vi "nanocal -- nuclear schottky fit V4.vi"() -> ()   [LabVIEW 2020] (continued)
              n311 = Number To Fractional String(number=w690, precision (6)=i16 3) -> (F-format string=w691:string)  [unwired: 2 in]
              n312 = Insert Into Map(map in=w694, key=w692, value=w690) -> (map out=w693:map{i32, dbl})  [unwired: 2 out]
            }
            "T lookup" <- w654
            n313 = for {
              shift-right: [w687] -> w649
              shift-left: w650 -> [w688]
              tunnel: [w685] -> w647 mode=indexing
              tunnel: w648 -> [w684] mode=indexing
              i -> [w686]
              n314 = Number To Decimal String(number=w684) -> (decimal integer string=w685:string)  [unwired: 1 in]
              n315 = Insert Into Map(map in=w688, key=w686, value=w684) -> (map out=w687:map{i32, dbl})  [unwired: 2 out]
            }
            "Side lookup" <- w649
            n316 = local read "Set of Change"() -> (w644:set{dbl})
            n317 = property on="select side (8S|4R)" class="Ring (strict)"("Strings []"=w647) -> ()  [unwired: 2 in, 2 out]
            n318 = for {
              shift-right: [w682] -> w645
              shift-left: w646 -> [w683]
              tunnel: [w680] -> w643 mode=indexing
              tunnel: w644 -> [w679] mode=indexing
              i -> [w681]
              n319 = Number To Decimal String(number=w679) -> (decimal integer string=w680:string)  [unwired: 1 in]
              n320 = Insert Into Map(map in=w683, key=w681, value=w679) -> (map out=w682:map{i32, dbl})  [unwired: 2 out]
            }
            "change lookup" <- w645
            n321 = local read "temps&degs"() -> (w660:map{string, map{T5, dbl}})
            n322 = local read "X selector"() -> (w659:T5)
            n323 = property on="select T (K)" class="Ring (strict)"("Strings []"=w653) -> ()  [unwired: 2 in, 2 out]
            n324 = for {
              tunnel: [w715] -> w670 mode=indexing
              tunnel: [w719] -> w668 mode=indexing
              tunnel: [w716] -> w672 mode=indexing
              tunnel: w659 -> [w720]
              tunnel: w640 -> [w718] mode=indexing
              tunnel: w660 -> [w717]
              n325 = Unbundle(w718) -> (w715:string, w716:string)
              n326 = Look In Map(map=w717, key=w716) -> (value=w721:map{T5, dbl})  [unwired: 1 in, 1 out]
              n327 = Look In Map(map=w721, key=w720) -> (value=w719:dbl)  [unwired: 1 in, 1 out]
            }
            n328 = property on="select set (1T|2B)" class="Ring (strict)"("Strings []"=w643) -> ()  [unwired: 2 in, 2 out]
            n329 = local read "Set of θ's"() -> (w658:set{dbl})
            n330 = local read "Set of B's"() -> (w657:set{dbl})
            n331 = for {
              shift-right: [w707] -> w667
              shift-left: w662 -> [w708]
              tunnel: [w705] -> w666 mode=indexing
              tunnel: w657 -> [w704] mode=indexing
              i -> [w706]
              n332 = Number To Fractional String(number=w704, precision (6)=i16 3) -> (F-format string=w705:string)  [unwired: 2 in]
              n333 = Insert Into Map(map in=w708, key=w706, value=w704) -> (map out=w707:map{i32, dbl})  [unwired: 2 out]
            }
            "B lookup" <- w667
            n334 = for {
              shift-right: [w713] -> w665
              shift-left: w661 -> [w714]
              tunnel: [w711] -> w664 mode=indexing
              tunnel: w658 -> [w710] mode=indexing
              i -> [w712]
              n335 = Number To Fractional String(number=w710, precision (6)=i16 3) -> (F-format string=w711:string)  [unwired: 2 in]
              n336 = Insert Into Map(map in=w714, key=w712, value=w710) -> (map out=w713:map{i32, dbl})  [unwired: 2 out]
            }
            "θ lookup" <- w665
            n337 = call "array - sorted inexes.vi"("x"=w668) -> ("index array"=w669:i32[])  [unwired: 9 in, 1 out]
            n338 = property on="select B (T)" class="Ring (strict)"("Strings []"=w666) -> ()  [unwired: 2 in, 2 out]
            n339 = property on="select θ (deg)" class="Ring (strict)"("Strings []"=w664) -> ()  [unwired: 2 in, 2 out]
            n340 = for {
              tunnel: w669 -> [w699] mode=indexing
              tunnel: w670 -> [w702]
              tunnel: [w701] -> w671 mode=indexing
              tunnel: w672 -> [w700]
              shift-right: [w695] -> w673
              shift-left: w663 -> [w698]
              i -> [w697]
              n341 = Index Array(array=w702, index=w699) -> (element=w701:string)
              n342 = Index Array(array=w700, index=w699) -> (element=w696:string)
              n343 = Insert Into Map(map in=w698, key=w697, value=w696) -> (map out=w695:map{i32, string})  [unwired: 2 out]
            }
            "filesnames lookup" <- w673
            n344 = property on="filenames" class="Ring (strict)"("Strings []"=w671) -> ()  [unwired: 2 in, 2 out]
          }
          frame "action: update constrained file selector" {
            (unwired) ""
            w728 = map{i32, string} {}  # Size: 0
            n345 = local read "state of all selectors"() -> (w724:map{T5, map{bool, dbl}})
            n346 = local read "all short filenames"() -> (w725:map{string, string})
            n347 = local read "temps&degs"() -> (w726:map{string, map{T5, dbl}})
            n348 = for {
              tunnel: w725 -> [w738] mode=indexing
              tunnel: [w738] -> w727 mode=indexing if=w735
              shift-right: [w737] -> w723
              shift-left: w726 -> [w737]
              tunnel: w724 -> [w734]
              n349 = for {
                tunnel: [w750] -> w736 mode=indexing
                shift-right: [w745] -> _
                shift-left: w738 -> [w745]
                shift-right: [w744] -> _
                shift-left: w737 -> [w744]
                tunnel: w734 -> [w743] mode=indexing
                n350 = Unbundle(w745) -> ("event data"=w749:string)  [unwired: 1 out]
                n351 = Unbundle(w743) -> ("Plost: sweep window"=w742:T5, "map"=w741:map{bool, dbl})
                n352 = for {
                  tunnel: w741 -> [w753] mode=indexing
                  tunnel: [w752] -> w739
                  tunnel: [w751] -> w740
                  n353 = Unbundle(w753) -> ("ignore side !"=w752:bool, "number OUT"=w751:dbl)
                }
                n354 = Look In Map(map=w744, key=w749) -> (value=w748:map{T5, dbl})  [unwired: 1 in, 1 out]
                n355 = Look In Map(map=w748, key=w742) -> (value=w747:dbl)  [unwired: 1 in, 1 out]
                n356 = Equal?(x=w747, y=w740) -> (x = y?=w746:bool)
                n357 = Or(x=w739, y=w746) -> (x .or. y?=w750:bool)
              }
              n358 = And Array Elements(Boolean array=w736) -> (logical AND=w735:bool)
            }
            n359 = for {
              tunnel: [w768] -> w731 mode=indexing
              tunnel: [w766] -> w729 mode=indexing
              tunnel: [w763] -> w733 mode=indexing
              tunnel: w727 -> [w765] mode=indexing
              tunnel: w723 -> [w764]
              n360 = Unbundle(w765) -> ("event data"=w763:string, "file pattern"=w768:string)
              n361 = local read "X selector"() -> (w762:T5)
              n362 = Look In Map(map=w764, key=w763) -> (value=w767:map{T5, dbl})  [unwired: 1 in, 1 out]
              n363 = Look In Map(map=w767, key=w762) -> (value=w766:dbl)  [unwired: 1 in, 1 out]
            }
            n364 = call "array - sorted inexes.vi"("x"=w729) -> ("index array"=w730:i32[])  [unwired: 9 in, 1 out]
            n365 = for {
              tunnel: w730 -> [w758] mode=indexing
              tunnel: w731 -> [w761]
              tunnel: [w760] -> w732 mode=indexing
              tunnel: w733 -> [w759]
              shift-right: [w754] -> w722
              shift-left: w728 -> [w757]
              i -> [w756]
              n366 = Index Array(array=w761, index=w758) -> (element=w760:string)
              n367 = Index Array(array=w759, index=w758) -> (element=w755:string)
              n368 = Insert Into Map(map in=w757, key=w756, value=w755) -> (map out=w754:map{i32, string})  [unwired: 2 out]
            }
            "constrained filename lookup" <- w722
            n369 = property on="constrained filenames :|\\" class="Ring (strict)"("Strings []"=w732) -> ()  [unwired: 2 in, 2 out]
          }
          frame "action: constrained filenames select" {
            n370 = local read "constrained filename lookup"() -> (w771:map{i32, string})
            n371 = local read "constrained filenames :|\\"() -> (w772:u16)
            n372 = local read "all full filenames"() -> (w773:map{string, path})
            n373 = Look In Map(map=w771, key=w772) -> (value=w774:string)  [unwired: 1 in, 1 out]
            n374 = Look In Map(map=w773, key=w774) -> (value=w775:path)  [unwired: 1 in, 1 out]
            n375 = for {
              N: 1 -> [_]
              tunnel: w769 -> [w777]
              tunnel: w775 -> [w776]
              n376 = local write "Read from file"(w776) -> ()
              n377 = Generate User Event(user event=w777, event data cluster="action: read from file" ("event data")) -> ()  [unwired: 2 in, 2 out]
            }
          }
          frame "action: write mathematica string" {
            n378 = local read "mathematica thing"() -> (w783:map{string, map{T5, dbl}})
            n379 = local read "folder"() -> (w782:path)
            n380 = Build Path(base path=w782, name or relative path="temporarystring.txt") -> (appended path=w781:path)
            n381 = call "string parse mathematica list assosiated array -- V2.vi"("derivative"=3-lorentzian-heat-response_action."create string", "Map IN"=w783) -> ("string out"=w779:string)  [unwired: 8 in, 1 out]
            "string OUT" <- w779
            n382 = Write to Text File(file (use dialog)=w781, text=w779) -> ()  [unwired: 2 in, 3 out]
          }
          frame "action: replot colors" {
            # "all -- including kappa0"
            n383 = local read "state of all selectors string"() -> (w796:string)
            n384 = local read "state of all selectors"() -> (w812:map{T5, map{bool, dbl}})
            n385 = local read "new selector names"() -> (w793:map{T5, map{T11, string}})
            n386 = local read "mathematica thing"() -> (w817:map{string, map{T5, dbl}})
            n387 = local read "X selector"() -> (w786:T5)
            n388 = control-ref of="Plot:  colors"() -> (w788:refnum<vi>)
            n389 = case shown="\"T (K)\", Default" w786 {
              tunnel: ["B (T)" "T (K)"] -> w785
              frame "B (T)" {
              }
              frame "T (K)", Default {
              }
            }
            n390 = Look In Map(map=w793, key=w786) -> (value=w792:map{T11, string})  [unwired: 1 in, 1 out]
            n391 = Array Subset(array=w816, index=0, length=6 ("index")) -> (w814:T5[])
            n392 = Look In Map(map=w792, key=nameformattingitem."nameL") -> (value=w790:string)  [unwired: 1 in, 1 out]
            n393 = call "replace plot - plot ref - V2.vi"("Plot ref in"=w788, "text"=w785, "cursor action"=cursor_action."set Xlabel") -> ("Plot ref out"=w787:refnum<vi>)  [unwired: 13 in, 3 out]
            n394 = Concatenate Strings(w796, w790) -> (w811:string)
            n395 = for {
              tunnel: w817 -> [w856]
              tunnel: w786 -> [w851]
              tunnel: w814 -> [w839] mode=indexing
              tunnel: w812 -> [w852]
              tunnel: w793 -> [w843]
              shift-right: [w847] -> w803
              shift-left: w811 -> [w850]
              tunnel: w796 -> [w848]
              tunnel: [w844] -> w805 mode=indexing
              tunnel: w787 -> [w836]
              n396 = for {
                tunnel: w856 -> [w883] mode=indexing
                tunnel: w839 -> [w882]
                tunnel: [w881] -> w855 mode=indexing if=w875
                tunnel: [w880] -> w854 mode=indexing if=w875
                tunnel: w851 -> [w879]
                tunnel: w852 -> [w878]
                n397 = Unbundle(w883) -> ("Map"=w877:map{T5, dbl})  [unwired: 1 out]
                n398 = for {
                  tunnel: w878 -> [w892] mode=indexing
                  tunnel: w877 -> [w891]
                  tunnel: [w889] -> w876 mode=indexing
                  n399 = Unbundle(w892) -> ("Plost: sweep window"=w890:T5, "map"=w888:map{bool, dbl})
                  n400 = for {
                    tunnel: w888 -> [w895] mode=indexing
                    tunnel: [w894] -> w885
                    tunnel: [w893] -> w886
                    n401 = Unbundle(w895) -> ("ignore side !"=w894:bool, "number OUT"=w893:dbl)
                  }
                  n402 = Look In Map(map=w891, key=w890) -> (value=w887:dbl)  [unwired: 1 in, 1 out]
                  n403 = Equal?(x=w887, y=w886) -> (x = y?=w884:bool)
                  n404 = Or(x=w885, y=w884) -> (x .or. y?=w889:bool)
                }
                n405 = Look In Map(map=w877, key=w879) -> (value=w881:dbl)  [unwired: 1 in, 1 out]
                n406 = Look In Map(map=w877, key=w882) -> (value=w880:dbl)  [unwired: 1 in, 1 out]
                n407 = And Array Elements(Boolean array=w876) -> (logical AND=w875:bool)
              }
              n408 = Look In Map(map=w843, key=w839) -> (value=w841:map{T11, string})  [unwired: 1 in, 1 out]
              n409 = Look In Map(map=w841, key=nameformattingitem."nameL") -> (value=w840:string)  [unwired: 1 in, 1 out]
              n410 = call <vilib>:"Space Constant.vi"() -> ("String"=w849:string)
              n411 = Concatenate Strings(w850, w849, w848, w840) -> (w847:string)
              n412 = call "array - sorted inexes.vi"("x"=w855) -> ("index array"=w853:i32[])  [unwired: 9 in, 1 out]
              n413 = local read "cursor index map"() -> (w837:map{T5, i32})
              n414 = for {
                tunnel: w855 -> [w874]
                tunnel: w854 -> [w873]
                tunnel: w853 -> [w870] mode=indexing
                tunnel: [w872] -> w846 mode=indexing
                tunnel: [w871] -> w845 mode=indexing
                n415 = Index Array(array=w874, index=w870) -> (element=w872:dbl)
                n416 = Index Array(array=w873, index=w870) -> (element=w871:dbl)
              }
              n417 = local read "color Map"() -> (w838:map{T5, u32})
              n418 = case shown="\"ζ\"..\"τC\", Default" w839 {
                selector: w839 -> [_ w865]
                tunnel: w846 -> [_ w867]
                tunnel: w845 -> [_ w866]
                tunnel: w838 -> [_ w864]
                tunnel: w837 -> [_ w863]
                tunnel: w836 -> [_ w862]
                frame "κ0" {
                }
                frame "ζ".."τC", Default {
                  n419 = Look In Map(map=w863, key=w865) -> (value=w858:i32)  [unwired: 1 in, 1 out]
                  n420 = Look In Map(map=w864, key=w865) -> (value=w857:u32)  [unwired: 1 in, 1 out]
                  n421 = call "replace plot - plot ref - V2.vi"("Plot ref in"=w862, "Array X IN"=w867, "Array Y IN"=w866, "plot index"=w858, "cursor action"=cursor_action."write") -> ("Plot ref out"=w861:refnum<vi>)  [unwired: 11 in, 3 out]
                  n422 = call "replace cursor - plot ref - V2.vi"("Plot ref in"=w861, "cursor index"=w858, "cursor action"=cursor_action."set cursor color", "Color Box"=w857) -> ("Plot ref out"=w860:refnum<vi>)  [unwired: 12 in, 3 out]
                  n423 = call "replace plot - plot ref - V2.vi"("Plot ref in"=w860, "plot index"=w858, "cursor action"=cursor_action."set plot color", "Color Box"=w857) -> ()  [unwired: 12 in, 4 out]
                }
              }
              n424 = Bundle(w846, w845) -> (w844:cluster{dbl[], dbl[]})  [unwired: 1 in]
            }
            n425 = Index Array(array=w805, index=0) -> (element=w809:cluster{dbl[], dbl[]})
            n426 = Unbundle(w809) -> (w808:dbl[])  [unwired: 1 out]
            n427 = Build Array(w808) -> (w807:dbl[][])
            n428 = for {
              shift-right: [w833] -> w806
              shift-left: w807 -> [w835]
              tunnel: w805 -> [w832] mode=indexing
              n429 = Unbundle(w832) -> (w834:dbl[])  [unwired: 1 out]
              n430 = Build Array (concatenate)(w835, w834) -> (w833:dbl[][])
            }
            n431 = local read "folder"() -> (w800:path)
            n432 = Concatenate Strings("plotstring", w796, ".dat") -> (w794:string)
            n433 = Concatenate Strings(w803, "\r") -> (w801:string)
            n434 = Transpose 2D Array(2D array=w806) -> (transposed array=w804:dbl[][])
            n435 = for {
              shift-right: [w825] -> w798
              shift-left: w801 -> [w824]
              tunnel: w804 -> [w822] mode=indexing
              n436 = for {
                shift-right: [w826] -> w821
                shift-left: "" -> [w831]
                tunnel: w822 -> [w830] mode=indexing
                n437 = Number To Fractional String(number=w830, precision (6)=i16 16) -> (F-format string=w828:string)  [unwired: 2 in]
                n438 = Concatenate Strings(w831, w828, "    ") -> (w826:string)
              }
              n439 = Concatenate Strings(w824, w821, "\r") -> (w825:string)
            }
            n440 = Build Path(base path=w800, name or relative path=w794) -> (appended path=w799:path)
            n441 = Write to Text File(file (use dialog)=w799, text=w798) -> ()  [unwired: 2 in, 3 out]
          }
          frame "action: update state of selectors" {
            w899 = T5[] [enum."T (K)", enum."B (T)", enum."θ (deg)", enum."side (S|R)"] items=["ζ", "τ1", "τS", "τN", "τC", "κ0", "m1", "m2", "m3", "T (K)", "B (T)", "θ (deg)", "side (S|R)", "change (B|T)"]
            n442 = local read "side map from NUM"() -> (w896:map{i32, T14})
            n443 = local read "select set (1T|2B)"() -> (w910:i32)
            n444 = local read "select side (8S|4R)"() -> (w929:i32)
            n445 = local read "ignore change !"() -> (w912:bool)
            n446 = Generate User Event(user event=w904, event data cluster="action: replot colors" ("event data")) -> (user event out=w905:refnum<user-event>)  [unwired: 2 in, 1 out]
            n447 = local read "change lookup"() -> (w911:map{i32, dbl})
            n448 = local read "select θ (deg)"() -> (w935:u16)
            n449 = local read "ignore side !"() -> (w926:bool)
            n450 = local read "Side lookup"() -> (w930:map{i32, dbl})
            n451 = local read "select T (K)"() -> (w931:u16)
            n452 = local read "select B (T)"() -> (w933:u16)
            n453 = local read "ignore B !"() -> (w920:bool)
            n454 = local read "ignore T !"() -> (w925:bool)
            n455 = local read "ignore θ !"() -> (w917:bool)
            n456 = local read "T lookup"() -> (w932:map{i32, dbl})
            n457 = local read "B lookup"() -> (w934:map{i32, dbl})
            n458 = local read "θ lookup"() -> (w936:map{i32, dbl})
            n459 = Look In Map(map=w934, key=w933) -> (value=w919:dbl)  [unwired: 1 in, 1 out]
            n460 = Look In Map(map=w932, key=w931) -> (value=w924:dbl)  [unwired: 1 in, 1 out]
            n461 = Look In Map(map=w936, key=w935) -> (value=w916:dbl)  [unwired: 1 in, 1 out]
            n462 = Look In Map(map=w930, key=w929) -> (value=w898:dbl)  [unwired: 1 in, 1 out]
            n463 = Look In Map(map=w911, key=w910) -> (value=w913:dbl)  [unwired: 1 in, 1 out]
            n464 = Generate User Event(user event=w905, event data cluster="action: update constrained file selector" ("event data")) -> ()  [unwired: 2 in, 2 out]
            n465 = node(w920, w919) -> (w918:map{bool, dbl})
            n466 = node(w925, w924) -> (w922:map{bool, dbl})
            n467 = node(w926, w898) -> (w927:map{bool, dbl})
            n468 = node(w917, w916) -> (w914:map{bool, dbl})
            n469 = Look In Map(map=w896, key=w898) -> (value=w897:T14)  [unwired: 1 in, 1 out]
            n470 = node(w912, w913) -> (w908:map{bool, dbl})
            n471 = local write "side"(w897) -> ()
            n472 = local read "new selector names"() -> (w902:map{T5, map{T11, string}})
            n473 = node(3-lorentzian-parameters."side (S|R)" ("Plost: sweep window"), w927, 3-lorentzian-parameters."T (K)" ("Plost: sweep window"), w922, 3-lorentzian-parameters."B (T)" ("Plost: sweep window"), w918, 3-lorentzian-parameters."θ (deg)" ("Plost: sweep window"), w914, 3-lorentzian-parameters."change (B|T)" ("Plost: sweep window"), w908) -> (w903:map{T5, map{bool, dbl}})
            "state of all selectors" <- w903
            n474 = for {
              shift-right: [w943] -> _
              shift-left: w903 -> [w943]
              tunnel: w902 -> [w939]
              shift-right: [w942] -> w900
              shift-left: "_" ("event data") -> [w941]
              tunnel: w899 -> [w938] mode=indexing
              n475 = Look In Map(map=w943, key=w938) -> (value=w945:map{bool, dbl})  [unwired: 1 in, 1 out]
              n476 = Look In Map(map=w939, key=w938) -> (value=w937:map{T11, string})  [unwired: 1 in, 1 out]
              n477 = for {
                tunnel: w945 -> [w960] mode=indexing
                tunnel: [w959] -> w944
                tunnel: [w958] -> w940
                n478 = Unbundle(w960) -> ("ignore side !"=w959:bool, "number OUT"=w958:dbl)
              }
              n479 = case shown="False" w944 {
                tunnel: [w956 w957] -> w942
                tunnel: w941 -> [w955 w957]
                tunnel: w940 -> [w952 _]
                tunnel: w937 -> [w948 _]
                frame False {
                  n480 = Look In Map(map=w948, key=nameformattingitem."prec") -> (value=w946:string)  [unwired: 1 in, 1 out]
                  n481 = Look In Map(map=w948, key=nameformattingitem."units") -> (value=w949:string)  [unwired: 1 in, 1 out]
                  n482 = Format Value(format string=w946, value (0)=w952) -> (output string=w951:string)  [unwired: 1 in]
                  n483 = Concatenate Strings(w955, "_" ("event data"), w951, w949, "_" ("event data")) -> (w956:string)
                }
                frame True {
                }
              }
            }
            "state of all selectors string" <- w900
          }
          frame "action: reset colors" {
            w967 = map{T5, u32} {}  # Size: 0
            n484 = local read "parameter"() -> (w974:T5[])
            n485 = local read "colors"() -> (w976:u32[])
            n486 = for {
              shift-right: [w979] -> w975
              shift-left: w967 -> [w980]
              tunnel: w974 -> [w978] mode=indexing
              tunnel: w976 -> [w977] mode=indexing
              n487 = Insert Into Map(map in=w980, key=w978, value=w977) -> (map out=w979:map{T5, u32})  [unwired: 2 out]
            }
            n488 = local write "color Map"(w975) -> ()
            n489 = Look In Map(map=w975, key=3-lorentzian-parameters."ζ" ("Plost: sweep window")) -> (value=w973:u32)  [unwired: 1 in, 1 out]
            n490 = Look In Map(map=w975, key=3-lorentzian-parameters."τ1" ("Plost: sweep window")) -> (value=w972:u32)  [unwired: 1 in, 1 out]
            n491 = Look In Map(map=w975, key=3-lorentzian-parameters."τS" ("Plost: sweep window")) -> (value=w971:u32)  [unwired: 1 in, 1 out]
            n492 = Look In Map(map=w975, key=3-lorentzian-parameters."τN" ("Plost: sweep window")) -> (value=w970:u32)  [unwired: 1 in, 1 out]
            n493 = Look In Map(map=w975, key=3-lorentzian-parameters."τC" ("Plost: sweep window")) -> (value=w969:u32)  [unwired: 1 in, 1 out]
            n494 = Look In Map(map=w975, key=3-lorentzian-parameters."κ0" ("Plost: sweep window")) -> (value=w968:u32)  [unwired: 1 in, 1 out]
            n495 = property on="ζ" class="Slide (strict)"("Fill Color"=w973) -> ()  [unwired: 2 in, 2 out]
            n496 = property on="T1" class="Slide (strict)"("Fill Color"=w972) -> ()  [unwired: 2 in, 2 out]
            n497 = property on="τS" class="Slide (strict)"("Fill Color"=w971) -> ()  [unwired: 2 in, 2 out]
            n498 = property on="τN" class="Slide (strict)"("Fill Color"=w970) -> ()  [unwired: 2 in, 2 out]
            n499 = property on="τC" class="Slide (strict)"("Fill Color"=w969) -> ()  [unwired: 2 in, 2 out]
            n500 = property on="κ0" class="Slide (strict)"("Fill Color"=w968) -> ()  [unwired: 2 in, 2 out]
          }
          frame "action: copy from math" {
            (unwired) 3-lorentzian-heat-response_action."dζ" ("derivative")
            n501 = local read "mathematica thing"() -> (w986:map{string, map{T5, dbl}})
            n502 = local read "key"() -> (w985:string)
            n503 = Generate User Event(user event=w981, event data cluster="action: new sweep" ("event data")) -> ()  [unwired: 2 in, 2 out]
            n504 = Look In Map(map=w986, key=w985) -> (key not found?=w983:bool, value=w984:map{T5, dbl})  [unwired: 1 in]
            n505 = case shown="False" w983 {
              tunnel: w984 -> [w992 _]
              frame False {
                n506 = Look In Map(map=w992, key=3-lorentzian-parameters."ζ" ("Plost: sweep window")) -> (value=w993:dbl)  [unwired: 1 in, 1 out]
                n507 = Look In Map(map=w992, key=3-lorentzian-parameters."τ1" ("Plost: sweep window")) -> (value=w991:dbl)  [unwired: 1 in, 1 out]
                n508 = Look In Map(map=w992, key=3-lorentzian-parameters."τS" ("Plost: sweep window")) -> (value=w990:dbl)  [unwired: 1 in, 1 out]
                n509 = Look In Map(map=w992, key=3-lorentzian-parameters."τN" ("Plost: sweep window")) -> (value=w989:dbl)  [unwired: 1 in, 1 out]
                n510 = Look In Map(map=w992, key=3-lorentzian-parameters."τC" ("Plost: sweep window")) -> (value=w988:dbl)  [unwired: 1 in, 1 out]
                n511 = Look In Map(map=w992, key=3-lorentzian-parameters."κ0" ("Plost: sweep window")) -> (value=w987:dbl)  [unwired: 1 in, 1 out]
                n512 = local write "ζ"(w993) -> ()
                n513 = local write "T1"(w991) -> ()
                n514 = local write "τS"(w990) -> ()
                n515 = local write "τN"(w989) -> ()
                n516 = local write "τC"(w988) -> ()
                n517 = local write "κ0"(w987) -> ()
              }
              frame True {
              }
            }
          }
          frame "action: copy to math" {
            w1010 = 0.0
            w1005 = T5[] [enum."ζ", enum."τ1", enum."τS", enum."τN", enum."τC", enum."κ0", enum."m1", enum."m2", enum."m3", enum."T (K)", enum."B (T)", enum."θ (deg)"] items=["ζ", "τ1", "τS", "τN", "τC", "κ0", "m1", "m2", "m3", "T (K)", "B (T)", "θ (deg)", "side (S|R)", "change (B|T)"]
            n518 = Generate User Event(user event=w1020, event data cluster="action: replot colors" ("event data")) -> ()  [unwired: 2 in, 2 out]
            n519 = local read "ζ"() -> (w1019:dbl)
            n520 = local read "T1"() -> (w1018:dbl)
            n521 = local read "τS"() -> (w1017:dbl)
            n522 = local read "τN"() -> (w1016:dbl)
            n523 = local read "τC"() -> (w1015:dbl)
            n524 = local read "κ0"() -> (w1014:dbl)
            n525 = local read "T (K)"() -> (w1009:dbl)
            n526 = local read "B (T)"() -> (w1008:dbl)
            n527 = local read "θ (deg)"() -> (w1007:dbl)
            n528 = Build Array(w1019, w1018, w1017, w1016, w1015, w1014, w1010, w1010, w1010, w1009, w1008, w1007) -> (w1006:dbl[])
            n529 = for {
              tunnel: w1006 -> [w1022] mode=indexing
              tunnel: w1005 -> [w1023] mode=indexing
              tunnel: [w1023] -> w1004 mode=indexing
              shift-right: [w1024] -> w1002
              shift-left: map{T5, dbl} {} ("Map") -> [w1025]
              n530 = Insert Into Map(map in=w1025, key=w1023, value=w1022) -> (map out=w1024:map{T5, dbl})  [unwired: 2 out]
            }
            n531 = local read "mathematica thing"() -> (w1013:map{string, map{T5, dbl}})
            n532 = local read "key"() -> (w1012:string)
            n533 = call "3-lorentzian-heat-response -- V4.vi"("action"=3-lorentzian-heat-response_action."calc m1m2m3", "Map IN"=w1002) -> ("Map OUT"=w1001:map{T5, dbl})  [unwired: 7 in, 2 out]
            n534 = in-place {
              in-place-border: w1004 -> [w1030]
              in-place-border: w1001 -> [w1026]
              n535 = in-place-map #2(w1013, w1012) -> (w1029:map{T5, dbl})  [unwired: 1 in, 1 out]
              n536 = for {
                tunnel: w1030 -> [w1032] mode=indexing
                shift-right: [w1034] -> w1028
                shift-left: w1029 -> [w1035]
                shift-right: [w1033] -> _
                shift-left: w1026 -> [w1033]
                n537 = Look In Map(map=w1033, key=w1032) -> (value=w1031:dbl)  [unwired: 1 in, 1 out]
                n538 = Insert Into Map(map in=w1035, key=w1032, value=w1031) -> (map out=w1034:map{T5, dbl})  [unwired: 2 out]
              }
              n539 = in-place-map #2(w1028, LVMapReplaceAction."Modify Entry only if found" ("action")) -> (w1011:map{string, map{T5, dbl}})  [unwired: 2 out]
            }
            n540 = local write "mathematica thing"(w1011) -> ()
          }
          frame "action: exit" {
          }
          frame "action: read from file" {
            n541 = local read "Read from file"() -> (w1037:path)
            n542 = Generate User Event(user event=w1077, event data cluster="action: new sweep" ("event data")) -> ()  [unwired: 2 in, 2 out]
            n543 = Unbundle("offset Re\noffset Im") -> ("Numeric"=w1062:dbl, "Numeric"=w1061:dbl)
            n544 = Re/Im To Complex(1:w1061, 2:w1062) -> (0:w1049:cdb)
            n545 = call "file - read-write - list of lines-V2.vi"("read/write control"=file_--_read-write_control."read", "file path"=w1037) -> ("header OUT"=w1046:string, "list of lines OUT"=w1048:string[], "filename out"=w1076:string)  [unwired: 7 in]
            n546 = call "filename-manage.vi"("filename-action"=filename-action."get name", "file name IN"=w1076) -> ("string OUT"=w1045:string)  [unwired: 7 in, 2 out]
            n547 = local read "cursor x selector"() -> (w1059:map{T5, dbl})
            n548 = case shown="\"raw nanocal\"" "data file formatting" {
              tunnel: [w1082 w1100 w1136 w1163] -> w1070
              tunnel: [w1081 w1099 w1135 w1162] -> w1064
              tunnel: w1049 -> [w1080 w1102 w1131 w1152]
              tunnel: w1048 -> [w1083 w1110 w1130 w1151]
              tunnel: w1046 -> [_ w1111 _ _]
              tunnel: w1045 -> [_ w1097 _ _]
              tunnel: w1037 -> [_ w1101 _ _]
              tunnel: "side" -> [_ w1096 _ _]
              frame "as is", Default {
                n549 = for {
                  tunnel: w1083 -> [w1094] mode=indexing
                  tunnel: [w1089] -> w1084 mode=indexing if=w1085
                  tunnel: [w1088] -> w1082 mode=indexing if=w1085
                  w1090 = 0.0
                  n550 = Scan From String(format string="%f%f%f", input string=w1094, initial scan location=u32 0, default 1=w1090, default 2=w1090, default 3=w1090) -> (offset past scan=w1086:u32, output 1=w1088:dbl, output 2=w1092:dbl, output 3=w1091:dbl)  [unwired: 1 in, 2 out]
                  n551 = Greater Than 0?(x=w1086) -> (x > 0?=w1085:bool)
                  n552 = Re/Im To Complex(1:w1091, 2:w1092) -> (0:w1089:cdb)
                }
                n553 = Subtract(x=w1084, y=w1080) -> (x-y=w1081:cdb[])
              }
              frame "raw nanocal" {
                n554 = case shown="\"ref\"" w1096 {
                  tunnel: [nanocal_raw_file_manage_action_V1."read S side" ("action") nanocal_raw_file_manage_action_V1."read R side" ("action")] -> w1095
                  frame "sam", Default {
                  }
                  frame "ref" {
                  }
                }
                n555 = call "nanocal_raw_file_manage_V1.vi"("action"=w1095, "list of lines IN"=w1110, "header IN"=w1111) -> ("z (K/W)  OUT"=w1103:cdb[], "f (Hz) OUT"=w1104:dbl[])  [unwired: 6 in, 1 out]
                n556 = Subtract(x=w1103, y=w1102) -> (x-y=w1105:cdb[])
                n557 = call "array -- freq-voltage transformations.vi"("freq voltage action"=array_--_freq-voltage_transformations_action."add -ω", "z In"=w1105, "ω IN"=w1104) -> ("z out"=w1108:cdb[], "ω out"=w1109:dbl[])  [unwired: 5 in, 2 out]
                n558 = call "array -- freq-voltage transformations.vi"("freq voltage action"=array_--_freq-voltage_transformations_action."sort ω", "z In"=w1108, "ω IN"=w1109) -> ("z out"=w1099:cdb[], "ω out"=w1100:dbl[])  [unwired: 5 in, 2 out]
                n559 = case shown="True" "toggle generate labview files" {
                  tunnel: w1101 -> [_ w1123]
                  tunnel: w1097 -> [_ w1127]
                  tunnel: w1100 -> [_ w1119]
                  tunnel: w1099 -> [_ w1118]
                  frame False {
                  }
                  frame True {
                    n560 = call "filename-manage.vi"("filename-action"=filename-action."get basename", "file name IN"=w1127) -> ("string OUT"=w1125:string)  [unwired: 7 in, 2 out]
                    n561 = Concatenate Strings(w1125, "_labview_.dat") -> (w1114:string)
                    n562 = Strip Path(path=w1123) -> (stripped path=w1122:path)  [unwired: 1 out]
                    n563 = call "array -- freq-voltage transformations.vi"("freq voltage action"=array_--_freq-voltage_transformations_action."labview file str", "z In"=w1118, "ω IN"=w1119) -> ("lines out"=w1116:string[], "header OUT"=w1117:string)  [unwired: 5 in, 2 out]
                    n564 = Build Path(base path=w1122, name or relative path=w1114) -> (appended path=w1121:path)
                    n565 = call "file - read-write - list of lines-V2.vi"("read/write control"=file_--_read-write_control."write all", "header IN"=w1117, "list of lines IN"=w1116, "file path"=w1121) -> ()  [unwired: 5 in, 3 out]
                  }
                }
              }
              frame "add - ω" {
                n566 = for {
                  tunnel: w1130 -> [w1148] mode=indexing
                  tunnel: [w1143] -> w1132 mode=indexing if=w1139
                  tunnel: [w1142] -> w1128 mode=indexing if=w1139
                  w1144 = 0.0
                  n567 = Scan From String(format string="%f%f%f", input string=w1148, initial scan location=u32 0, default 1=w1144, default 2=w1144, default 3=w1144) -> (offset past scan=w1140:u32, output 1=w1142:dbl, output 2=w1146:dbl, output 3=w1145:dbl)  [unwired: 1 in, 2 out]
                  n568 = Greater Than 0?(x=w1140) -> (x > 0?=w1139:bool)
                  n569 = Re/Im To Complex(1:w1145, 2:w1146) -> (0:w1143:cdb)
                }
                n570 = Subtract(x=w1132, y=w1131) -> (x-y=w1129:cdb[])
                n571 = call "array -- freq-voltage transformations.vi"("freq voltage action"=array_--_freq-voltage_transformations_action."add -ω", "z In"=w1129, "ω IN"=w1128) -> ("z out"=w1137:cdb[], "ω out"=w1138:dbl[])  [unwired: 5 in, 2 out]
                n572 = call "array -- freq-voltage transformations.vi"("freq voltage action"=array_--_freq-voltage_transformations_action."sort ω", "z In"=w1137, "ω IN"=w1138) -> ("z out"=w1135:cdb[], "ω out"=w1136:dbl[])  [unwired: 5 in, 2 out]
              }
              frame "full rydh" {
                n573 = for {
                  tunnel: w1151 -> [w1175] mode=indexing
                  tunnel: [w1170] -> w1153 mode=indexing if=w1166
                  tunnel: [w1169] -> w1149 mode=indexing if=w1166
                  w1171 = 0.0
                  n574 = Scan From String(format string="%f%f%f", input string=w1175, initial scan location=u32 0, default 1=w1171, default 2=w1171, default 3=w1171) -> (offset past scan=w1167:u32, output 1=w1169:dbl, output 2=w1173:dbl, output 3=w1172:dbl)  [unwired: 1 in, 2 out]
                  n575 = Greater Than 0?(x=w1167) -> (x > 0?=w1166:bool)
                  n576 = Re/Im To Complex(1:w1172, 2:w1173) -> (0:w1170:cdb)
                }
                n577 = Subtract(x=w1153, y=w1152) -> (x-y=w1150:cdb[])
                n578 = call "array -- freq-voltage transformations.vi"("freq voltage action"=array_--_freq-voltage_transformations_action."2 x ω", "z In"=w1150, "ω IN"=w1149) -> ("z out"=w1157:cdb[], "ω out"=w1159:dbl[])  [unwired: 5 in, 2 out]
                n579 = call "array -- freq-voltage transformations.vi"("freq voltage action"=array_--_freq-voltage_transformations_action."R-phase(deg) to Re-Im", "z In"=w1157, "ω IN"=w1159) -> ("z out"=w1156:cdb[], "ω out"=w1158:dbl[])  [unwired: 5 in, 2 out]
                n580 = call "array -- freq-voltage transformations.vi"("freq voltage action"=array_--_freq-voltage_transformations_action."add -ω", "z In"=w1156, "ω IN"=w1158) -> ("z out"=w1164:cdb[], "ω out"=w1165:dbl[])  [unwired: 5 in, 2 out]
                n581 = call "array -- freq-voltage transformations.vi"("freq voltage action"=array_--_freq-voltage_transformations_action."sort ω", "z In"=w1164, "ω IN"=w1165) -> ("z out"=w1162:cdb[], "ω out"=w1163:dbl[])  [unwired: 5 in, 2 out]
              }
            }
            n582 = call "filename-manage.vi"("filename-action"=filename-action."get T", "file name IN"=w1045) -> ("number OUT"=w1058:dbl, "filename OUT"=w1073:string)  [unwired: 7 in, 1 out]
            "T (K)" <- w1058
            n583 = Insert Into Map(map in=w1059, key=3-lorentzian-parameters."T (K)" ("Plost: sweep window"), value=w1058) -> (map out=w1057:map{T5, dbl})  [unwired: 2 out]
            n584 = call "filename-manage.vi"("filename-action"=filename-action."get deg", "file name IN"=w1073) -> ("number OUT"=w1054:dbl, "filename OUT"=w1040:string)  [unwired: 7 in, 1 out]
            "θ (deg)" <- w1054
            n585 = Insert Into Map(map in=w1057, key=3-lorentzian-parameters."θ (deg)" ("Plost: sweep window"), value=w1054) -> (map out=w1056:map{T5, dbl})  [unwired: 2 out]
            n586 = call "filename-manage.vi"("filename-action"=filename-action."get B", "file name IN"=w1040) -> ("number OUT"=w1053:dbl, "filename OUT"=w1039:string)  [unwired: 7 in, 1 out]
            "B (T)" <- w1053
            n587 = Insert Into Map(map in=w1056, key=3-lorentzian-parameters."B (T)" ("Plost: sweep window"), value=w1053) -> (map out=w1055:map{T5, dbl})  [unwired: 2 out]
            n588 = local write "cursor x selector"(w1055) -> ()
            n589 = local read "side map to STR"() -> (w1038:map{T14, string})
            n590 = call "filename-manage.vi"("filename-action"=filename-action."getIDStock", "file name IN"=w1039) -> ("string OUT"=w1043:string)  [unwired: 7 in, 2 out]
            "file IDS" <- w1043
            n591 = Look In Map(map=w1038, key="side") -> (value=w1044:string)  [unwired: 1 in, 1 out]
            n592 = Concatenate Strings(w1043, w1044) -> (→"key":string)
            n593 = call "filter - complex - four.vi"("omega (Hz) in"=w1070, "z in"=w1064, "span"="cspan") -> ("omega out"=w1069:dbl[], "z out"=w1068:cdb[], "dz/domega out"=w1067:cdb[])  [unwired: 9 in, 5 out]
            n594 = call "nanocal -- publish -- freq scan V2.vi"("publisher action"=publisher_action."set", "dz/dω IN (V)"=w1067, "z IN (V)"=w1068, "ω IN (Hz)"=w1069) -> ()  [unwired: 5 in, 3 out]
          }
          frame "action: save freq scan" {
            n595 = local read "Freq sweep name template"() -> (w1181:T6)
            n596 = call "MFLI -- publish -- freq scan.vi"("publisher action"=publisher_action."get") -> ("Voltage out (V)"=w1177:cdb[], "Freq out (Hz)"=w1178:dbl[])  [unwired: 9 in]
            n597 = call "filename-manage.vi"("filename pattern"=w1181, "filename-action"=filename-action."uniquenum", "folder IN"="Save folder", "file name IN"="freq sweep file name") -> ("filename OUT"=w1180:string)  [unwired: 5 in, 2 out]
            n598 = call "KM_appendline -- freq sweep.vi"("freq"=w1178, "Vout(V)"=w1177, "Save frequency scan"="Save folder", "read/write control"=KM_file_--_read-write_control."append one line", "name or relative path"=w1180) -> ()  [unwired: 15 in]
            n599 = local write "freq sweep file name"(w1180) -> ()
          }
          frame "void", Default {
          }
        }
      }
    }
  }
  n600 = local write "newton pause"(w34) -> ()
  n601 = control-ref of="Plot:  colors"() -> (w35:refnum<vi>)
  n602 = call "replace cursor - plot ref - V2.vi"("Plot ref in"=w38, "new X"=w37, "new  Y"=w37, "cursor index"=2, "cursor action"=cursor_action."write") -> ()  [unwired: 11 in, 4 out]
  n603 = while "interface" {
    tunnel: w52 -> [w1189]
    tunnel: w41 -> [w1188]
    tunnel: w38 -> [w1186]
    tunnel: w35 -> [w1185]
    tunnel: w34 -> [_]
    stop <- w1187 stop-if-true
    n604 = event shown="[13] Key Down" {
      selector: w1189 -> [_ _ _ _ _ _ _ _ _ _ _ _ _ _ _ _ _ _ _ _ _ _ _ _ _ _ _]
      dyn-events: _ -> [_ _ _ _ _ _ _ _ _ _ _ _ _ _ _ _ _ _ _ _ _ _ _ _ _ _ _]
      timeout: _ -> [_ _ _ _ _ _ _ _ _ _ _ _ _ _ _ _ _ _ _ _ _ _ _ _ _ _ _]
      tunnel: w1188 -> [w1190 _ w1202 w1204 _ w1233 w1235 w1238 w1243 w1245 w1247 w1249 w1252 w1258 w1324 _ w1352 w1355 w1358 w1361 w1364 w1367 w1375 w1379 _ w1427 w1430]
      tunnel: [_ _ _ _ _ _ _ _ "load! :l" _ _ _ _ _ _ _ _ _ _ _ _ _ _ _ _ _ _] -> _
      tunnel: [_ _ _ _ _ _ _ _ _ _ _ _ _ _ _ _ _ _ _ _ _ _ _ _ w1381 _ _] -> w1187
      tunnel: [_ _ _ _ _ "go!" _ _ _ _ _ _ "parse! :p" _ _ "pause!" "uco! :u" "read τ from Math ! :q" "write τ to Math! :p" "Math --> string OUT  ! :s" "generate empty string from filelist !" "string IN  --> Math!" _ _ _ "plot landscape!" _] -> _
      tunnel: w1186 -> [_ _ _ _ _ _ _ _ _ _ _ _ _ w1254 _ _ _ _ _ _ _ _ _ _ _ _ _]
      tunnel: w1185 -> [_ _ _ _ _ _ _ _ _ _ _ _ _ _ w1347 _ _ _ _ _ _ _ _ _ _ _ _]
      tunnel: [_ _ _ _ _ _ _ _ _ "Read from file" _ _ _ _ _ _ _ _ _ _ _ _ _ _ _ _ _] -> _
      event "Plot: sweep window": Cursor Move {
        n605 = event-data() -> ("CursIdx"=w1191:i32)  [unwired: 1 in]
        n606 = case shown="0..2" w1191 {
          tunnel: w1190 -> [w1193 _]
          frame 0..2 {
            w1192 = "action: fit"  # action
            n607 = Generate User Event(user event=w1193, event data cluster=w1192) -> ()  [unwired: 2 in, 2 out]
          }
          frame 3..5, Default {
          }
        }
      }
      event "scale gauge: Plot: complex plane": Value Change {
        n608 = event-data() -> ()  [unwired: 1 in, 1 out]
        n609 = local read "scale gauge: Plot: complex plane"() -> (w1200:dbl)
        n610 = control-ref of="Plot: sweep window"() -> (w1199:refnum<vi>)
        n611 = Multiply(x=w1200, y=0.3) -> (x*y=w1201:dbl)
        n612 = Bundle By Name(cluster=T30 {"window y"=0.0021014740628288917, "center x"=44850.89441339177, "center y"=2.5658109925320947, "window x"=17480.201988350764} ("window IN"), "window x"=w1200, "window y"=w1200, "center x"=w1201, "center y"=0.0) -> (w1198:T30)
        n613 = call "replace cursor - plot ref - V2.vi"("Plot ref in"=w1199, "window IN"=w1198, "cursor action"=cursor_action."zoom to win") -> ()  [unwired: 13 in, 4 out]
      }
      event "ζ", "T1", "τS", "τN", "τC", "κ0": Value Change {
        n614 = event-data() -> ()  [unwired: 1 in, 1 out]
        n615 = Generate User Event(user event=w1202, event data cluster="action: new sweep" ("event data")) -> ()  [unwired: 2 in, 2 out]
      }
      event Value Change {
        n616 = event-data() -> ()  [unwired: 1 in, 6 out]
        n617 = Generate User Event(user event=w1204, event data cluster="action: update enums" ("event data")) -> ()  [unwired: 2 in, 2 out]
      }
      event "ω0 (rad/sec)": Value Change {
        n618 = event-data() -> ()  [unwired: 1 in, 1 out]
        n619 = call "nanocal -- publish -- freq scan V2.vi"("publisher action"=publisher_action."get") -> ("z out (V)"=w1231:cdb[], "ω out (Hz)"=w1226:dbl[])  [unwired: 8 in, 1 out]
        n620 = control-ref of="Plot: sweep window"() -> (w1213:refnum<vi>)
        n621 = local read "T1"() -> (w1215:dbl)
        n622 = local read "τN"() -> (w1217:dbl)
        n623 = local read "ζ"() -> (w1214:dbl)
        n624 = local read "τS"() -> (w1216:dbl)
        n625 = local read "τC"() -> (w1218:dbl)
        n626 = local read "κ0"() -> (w1219:dbl)
        n627 = Divide(x="ω0 (rad/sec)", y=6.283185307179586) -> (x/y=w1224:dbl)
        n628 = call "3-lorentzian-heat-response.vi"("zeta"=w1214, "T1"=w1215, "tauS"=w1216, "tauN"=w1217, "tauC"=w1218, "kappa0"=w1219, "omega (rad/sec)"="ω0 (rad/sec)", "action"=3-lorentzian-heat-response_action."calc R") -> ("Romega"=w1222:cdb)  [unwired: 7 in, 4 out]
        n629 = Complex To Re/Im(x + iy=w1222) -> (x=w1220:dbl, y=w1221:dbl)
        n630 = Threshold 1D Array(2:w1224, 3:w1226) -> (0:w1225:dbl)  [unwired: 1 in]
        n631 = call "replace cursor - plot ref - V2.vi"("Plot ref in"=w1213, "new X"=w1220, "new  Y"=w1221, "cursor index"=0, "cursor action"=cursor_action."write") -> ("Plot ref out"=w1227:refnum<vi>)  [unwired: 11 in, 3 out]
        n632 = Index Array(array=w1231, index=w1225) -> (element=w1228:cdb)
        n633 = Complex To Re/Im(x + iy=w1228) -> (x=w1229:dbl, y=w1230:dbl)
        n634 = call "replace cursor - plot ref - V2.vi"("Plot ref in"=w1227, "new X"=w1229, "new  Y"=w1230, "cursor index"=1, "cursor action"=cursor_action."write") -> ()  [unwired: 11 in, 4 out]
      }
      event "go!": Value Change {
        n635 = event-data() -> ()  [unwired: 1 in, 6 out]
        n636 = Generate User Event(user event=w1233, event data cluster="action: gradient step" ("event data")) -> ()  [unwired: 2 in, 2 out]
      }
      event "select side (8S|4R)", "select θ (deg)", "ignore T !", "select T (K)", "ignore B !", "ignore θ !", "select B (T)", "ignore side !", "ignore change !", "select set (1T|2B)": Value Change {
        n637 = event-data() -> ()  [unwired: 1 in, 6 out]
        n638 = Generate User Event(user event=w1235, event data cluster="action: update state of selectors" ("event data")) -> ()  [unwired: 2 in, 2 out]
      }
      event "Plot: sweep window": Cursor Release {
        n639 = event-data() -> ("CursIdx"=w1237:i32)  [unwired: 1 in]
        n640 = case shown="0..2" w1237 {
          tunnel: w1238 -> [_ w1239]
          frame 3, Default {
          }
          frame 0..2 {
            w1240 = "action: fit"  # event data
            n641 = Generate User Event(user event=w1239, event data cluster=w1240) -> ()  [unwired: 2 in, 2 out]
          }
        }
      }
      event "load! :l": Value Change {
        n642 = event-data() -> ()  [unwired: 1 in, 6 out]
        n643 = Generate User Event "action User Event"(user event=w1243, event data cluster="action: read from file" ("event data")) -> ()  [unwired: 2 in, 2 out]
      }
      event "Read from file": Value Change {
